vi "Read.vi"(8 "error in (no error)":errorcluster, 11 "Configuration":refnum<class "Configuration.lvclass">) -> (0 "error out":errorcluster, 3 "Configuration out":refnum<class "Configuration.lvclass">)   [LabVIEW 2012, in "Configuration.lvlib" / "Configuration.lvclass"]
doc: "Read configuration data."
uses:
  Configuration.lvclass
  Configuration.lvclass/Configuration.ctl
  Interface/Interface.lvclass
  Section/Section.lvclass
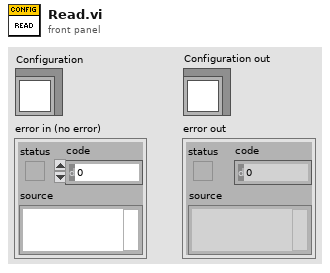
[diagram p1: front panel]
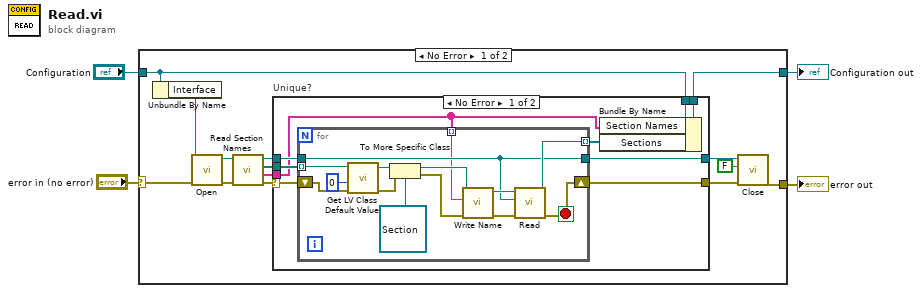
[diagram p0: block diagram]
diagram:
  n1 = case shown="No Error" "error in (no error)" {
    selector: "error in (no error)" -> [w13 w46]
    tunnel: [w5 w46] -> w3
    tunnel: [w18 w45] -> w2
    tunnel: "Configuration" -> [w11 w45]
    frame No Error {
      n2 = Unbundle By Name(w11) -> ("Interface"=w10:refnum<class "Interface.lvclass">)
      n3 = call-dynamic "Open.vi"("error in (no error)"=w13, "Interface in"=w10) -> ("error out"=w12:errorcluster, "Interface out"=w14:refnum<class "Interface.lvclass">)  [unwired: 8 in]
      n4 = call-dynamic "Read Section Names.vi"("error in (no error)"=w12, "Interface in"=w14) -> ("error out"=w9:errorcluster, "Section Names"=w16:string[], "Section Classes"=w17:path[], "Interface out"=w15:refnum<class "Interface.lvclass">)  [unwired: 6 in]
      n5 = case "Unique?" shown="No Error" w9 {
        selector: w9 -> [w22 w43]
        tunnel: w15 -> [w27 w42]
        tunnel: w11 -> [w26 w44]
        tunnel: [w25 w44] -> w18
        tunnel: [w19 w43] -> w6
        tunnel: w17 -> [w23 _]
        tunnel: w16 -> [w21 _]
        tunnel: [w20 w42] -> w7
        frame No Error {
          n6 = for {
            tunnel: w27 -> [w29]
            shift-right: [w32] -> w19
            shift-left: w22 -> [w41]
            tunnel: [w31] -> w24 mode=indexing
            tunnel: w23 -> [w30] mode=indexing
            tunnel: [w29] -> w20
            tunnel: w21 -> [w28] mode=indexing
            stop <- w32 stop-if-true
            n7 = call <vilib>:"Get LV Class Default Value.vi"("error in (no error)"=w41, "options"=u32 0, "class path"=w30) -> ("error out"=w39:errorcluster, "object"=w40:refnum<class>)  [unwired: 7 in]
            n8 = To More Specific Class(target class=refnum<class "Section.lvclass"> refnum ("LVOOP Introduction.lvlib:Section.lvclass"), reference=w40, error in=w39) -> (specific class reference=w37:refnum<class "Section.lvclass">, error out=w36:errorcluster)
            n9 = call "Write Name.vi"("error in (no error)"=w36, "Name"=w28, "Section in"=w37) -> ("error out"=w33:errorcluster, "Section out"=w34:refnum<class "Section.lvclass">)  [unwired: 7 in]
            n10 = call "Read.vi"("error in (no error)"=w33, "Interface"=w29, "Section in"=w34) -> ("error out"=w32:errorcluster, "Section out"=w31:refnum<class "Section.lvclass">)  [unwired: 7 in]
          }
          n11 = Bundle By Name(cluster=w26, "Section Names"=w21, "Sections"=w24) -> (w25:refnum<class "Configuration.lvclass">)
        }
        frame Error {
        }
      }
      n12 = call-dynamic "Close.vi"("error in (no error)"=w6, "write if changed (T)"=FALSE, "Interface in"=w7) -> ("error out"=w5:errorcluster)  [unwired: 7 in, 1 out]
    }
    frame Error {
    }
  }
  "error out" <- w3
  "Configuration out" <- w2
